vi "niFpga wdp fft DIT 4spc.vi"(0 "real data in":fxp<+/-,8,1>[](array[numeric])=[0.0, 0.0, 0.0, 0.0], 5 "imaginary data in":fxp<+/-,8,1>[](array[numeric])=[0.0, 0.0, 0.0, 0.0], 9 "input frame start":bool, 12 "enable":bool) -> (3 "data indices":u16[](array[numeric]), 4 "real data out":fxp<+,8,1>[](array[numeric]) format="%#.6g", 6 "imaginary data out":fxp<+,8,1>[](array[numeric]) format="%#.6g", 10 "output valid":bool, 14 "ready for frame":bool, 15 "output frame start":bool)   [LabVIEW 2017]
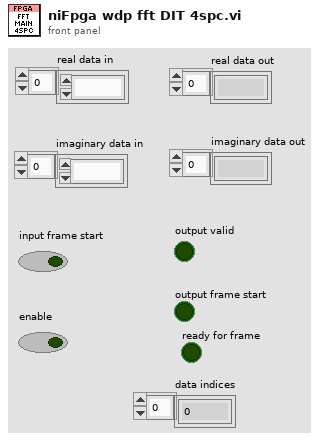
[diagram p1: front panel]
types:
  T1 = cluster{"internal input type":fxp<+/-,8,1>, "internal input type":fxp<+/-,8,1>}
  T2 = cluster{"twiddle factor type":fxp<+/-,16,2>, "twiddle factor type":fxp<+/-,16,2>}[]
  T3 = cluster{"x-y":fxp<+/-,19,12>, "x-y":fxp<+/-,19,12>}
  T4 = cluster{"x+y":fxp<+/-,19,12>, "x+y":fxp<+/-,19,12>}
  T5 = cluster{"x+y":fxp<+/-,19,12>, "x+y":fxp<+/-,19,12>}[]
  T6 = cluster{"x-y":fxp<+/-,19,12>, "x-y":fxp<+/-,19,12>}[]
  T7 = cluster{"data re":fxp<+/-,8,1>, "data im":fxp<+/-,8,1>}[]
  T8 = cluster{"x-y":fxp<+/-,20,13>, "x-y":fxp<+/-,20,13>}[]
  T9 = cluster{"x-y":fxp<+/-,20,13>, "x-y":fxp<+/-,20,13>}
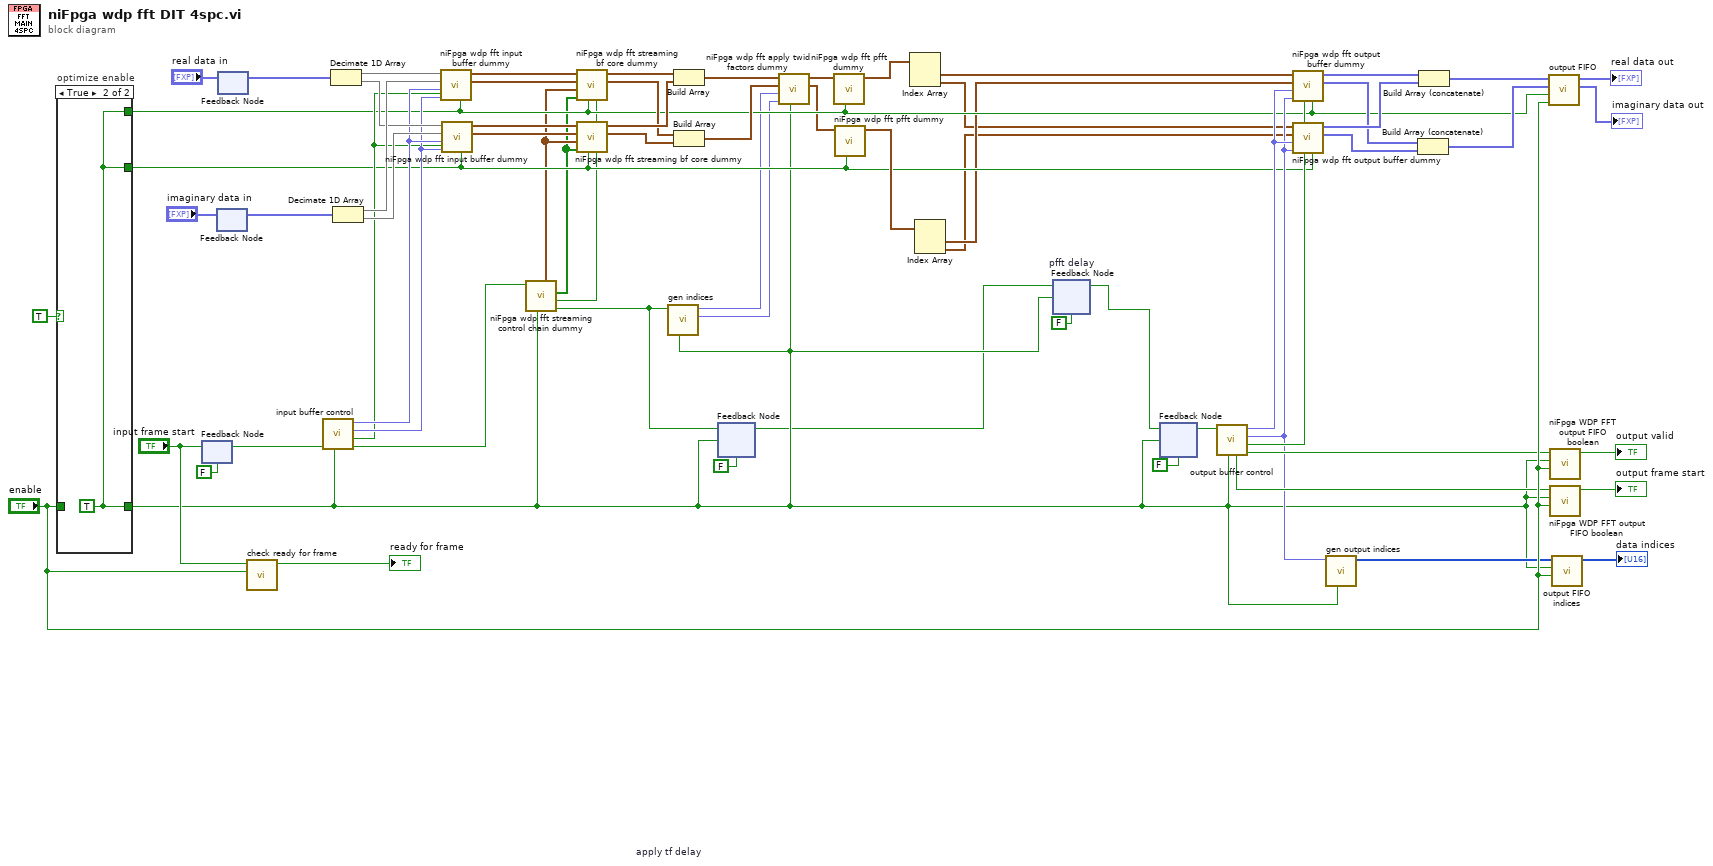
[diagram p0: block diagram]
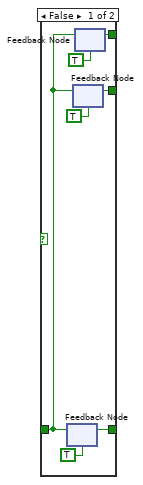
[diagram p2: hidden frame]
diagram:
  n1 = case "optimize enable" shown="True" TRUE {
    tunnel: [w73 w76] -> w10
    tunnel: "enable" -> [w71 _]
    tunnel: [w70 w76] -> w18
    tunnel: [w69 w76] -> w17
    frame False {
      n2 = feedback #1(TRUE ("enable")) -> (w73:bool)
      n3 = feedback-in #1(w71) -> ()
      n4 = feedback #2(TRUE ("enable")) -> (w69:bool)
      n5 = feedback-in #2(w71) -> ()
      n6 = feedback #3(TRUE ("enable")) -> (w70:bool)
      n7 = feedback-in #3(w71) -> ()
    }
    frame True {
      w76 = TRUE
    }
  }
  n8 = feedback #4(FALSE ("enable")) -> (w61:bool)
  n9 = feedback-in #4("input frame start") -> ()
  n10 = feedback #5() -> (w47:fxp<+/-,8,1>[])  [unwired: 1 in]
  n11 = feedback-in #5("imaginary data in") -> ()
  n12 = feedback #6() -> (w48:fxp<+/-,8,1>[])  [unwired: 1 in]
  n13 = feedback-in #6("real data in") -> ()
  n14 = call "check ready for frame"("enable"="enable", "frame start in"="input frame start") -> ("ready for frame"=→"ready for frame":bool)  [unwired: 9 in]
  n15 = call "input buffer control"("enable"=w10, "frame start in"=w61) -> ("frame start out"=w60:bool, "write memory 2?"=w31:bool, "read index"=w41:fxp<+,9,9>, "write index"=w42:fxp<+,8,8>)  [unwired: 6 in]
  n16 = Decimate 1D Array(w48) -> (w46:fxp<+/-,8,1>[], w44:fxp<+/-,8,1>[])
  n17 = Decimate 1D Array(w47) -> (w45:fxp<+/-,8,1>[], w43:fxp<+/-,8,1>[])
  n18 = call <vilib>:"niFpga wdp fft input buffer dummy.vi"("enable"=w18, "write memory 2?"=w31, "read index"=w41, "write index"=w42, "data in im"=w45, "data in re"=w46) -> ("data out 1"=w39:T1, "data out 0"=w40:T1)  [unwired: 4 in]
  n19 = call <vilib>:"niFpga wdp fft input buffer dummy.vi"("enable"=w17, "write memory 2?"=w31, "read index"=w41, "write index"=w42, "data in im"=w43, "data in re"=w44) -> ("data out 1"=w37:T1, "data out 0"=w38:T1)  [unwired: 4 in]
  n20 = call <vilib>:"niFpga wdp fft streaming control chain dummy.vi"("enable"=w10, "input frame start"=w60) -> ("frame start"=w19:bool, "index=0?"=w4:bool, "switch"=w5:bool[], "twiddle factors"=w6:T2)  [unwired: 5 in, 1 out]
  n21 = call <vilib>:"niFpga wdp fft streaming bf core dummy.vi"("index=0?"=w4, "enable"=w18, "switch"=w5, "twiddle factors"=w6, "data in 1"=w39, "data in 0"=w40) -> ("data out 1"=w56:T3, "data out 0"=w58:T4)  [unwired: 4 in]
  n22 = call <vilib>:"niFpga wdp fft streaming bf core dummy.vi"("index=0?"=w4, "enable"=w17, "switch"=w5, "twiddle factors"=w6, "data in 1"=w37, "data in 0"=w38) -> ("data out 1"=w55:T3, "data out 0"=w57:T4)  [unwired: 4 in]
  n23 = call "gen indices"("enable"=w10, "frame start"=w19) -> ("data index 1"=w8:fxp<+,10,10>, "data index 0"=w9:fxp<+,10,10>)  [unwired: 8 in]
  n24 = Build Array(w58, w57) -> (w54:T5)
  n25 = Build Array(w56, w55) -> (w53:T6)
  n26 = feedback #7 "apply tf delay"(FALSE) -> (w7:bool)
  n27 = feedback-in #7(w19, w10) -> ()
  n28 = call <vilib>:"niFpga wdp fft apply twid factors dummy.vi"("enable"=w10, "data index 1"=w8, "data index 0"=w9, "data in 1"=w53, "data in 0"=w54) -> ("data out 1"=w2:T7, "data out 0"=w3:T7)  [unwired: 5 in]
  n29 = call <vilib>:"niFpga wdp fft pfft dummy.vi"("enable"=w18, "data in"=w3) -> ("data out"=w68:T8)  [unwired: 9 in]
  n30 = call <vilib>:"niFpga wdp fft pfft dummy.vi"("enable"=w17, "data in"=w2) -> ("data out"=w67:T8)  [unwired: 9 in]
  n31 = Index Array(array=w68) -> (element #1=w16:T9, element #2=w14:T9)  [unwired: 2 in]
  n32 = Index Array(array=w67) -> (element #1=w15:T9, element #2=w13:T9)  [unwired: 2 in]
  n33 = feedback #8 "pfft delay"(FALSE) -> (w12:bool)
  n34 = feedback-in #8(w7, w10) -> ()
  n35 = feedback #9 ("delay")(FALSE) -> (w11:bool)
  n36 = feedback-in #9(w12, w10) -> ()
  n37 = call "output buffer control"("enable"=w10, "frame start"=w11) -> ("output valid?"=w26:bool, "memory switch"=w24:bool, "read index"=w23:fxp<+,4,4>, "write index"=w25:fxp<+,9,9>, "frame start?"=w27:bool)  [unwired: 5 in]
  n38 = call <vilib>:"niFpga wdp fft output buffer dummy.vi"("enable"=w18, "memory switch"=w24, "read index"=w23, "write index"=w25, "data in 1"=w15, "data in 0"=w16) -> ("data out im"=w50:fxp<+/-,32,16>[], "data out re"=w52:fxp<+/-,32,16>[])  [unwired: 4 in]
  n39 = call <vilib>:"niFpga wdp fft output buffer dummy.vi"("enable"=w17, "memory switch"=w24, "read index"=w23, "write index"=w25, "data in 1"=w13, "data in 0"=w14) -> ("data out im"=w49:fxp<+/-,32,16>[], "data out re"=w51:fxp<+/-,32,16>[])  [unwired: 4 in]
  n40 = call "gen output indices"("enable"=w10, "index"=w23) -> ("data indices"=w22:u16[])  [unwired: 9 in]
  n41 = Build Array (concatenate)(w50, w49) -> (w34:fxp<+/-,32,16>[])
  n42 = Build Array (concatenate)(w52, w51) -> (w35:fxp<+/-,32,16>[])
  n43 = call "output FIFO"("enable"="enable", "enable with delay"=w18, "data in 1"=w34, "data in 0"=w35) -> ("data out 1"=→"imaginary data out":fxp<+,8,1>[], "data out 0"=→"real data out":fxp<+,8,1>[])  [unwired: 6 in]
  n44 = call <vilib>:"niFpga WDP FFT output FIFO boolean.vi"("enable"="enable", "enable with delay"=w10, "boolean in"=w26) -> ("boolean out"=→"output valid":bool)  [unwired: 8 in]
  n45 = call <vilib>:"niFpga WDP FFT output FIFO boolean.vi"("enable"="enable", "enable with delay"=w10, "boolean in"=w27) -> ("boolean out"=→"output frame start":bool)  [unwired: 8 in]
  n46 = call "output FIFO indices"("enable"="enable", "enable with delay"=w10, "data in"=w22) -> ("data out"=→"data indices":u16[])  [unwired: 8 in]
